vi "WPI_SPIWrite.vi"(8 "error in (no error)":errorcluster, 10 "Data To Send":u8[](array[numeric]), 11 "SPIDevRef":T1) -> (0 "error out":errorcluster, 2 "Received Data":u8[](array[numeric]), 3 "SPIDevRef":T1)   [LabVIEW 2017]
doc: "Writes data to the slave device.\n\nThis software is licensed. Open the labview\\readme\\WPI Robotics Library Open Source License.txt file for more information."
uses:
  <vilib>/Rock Robotics/WPI/SPI/WPI_SPIDevRef.ctl
  <vilib>/Rock Robotics/SystemInterfaces/spilib/spi_bus.ctl
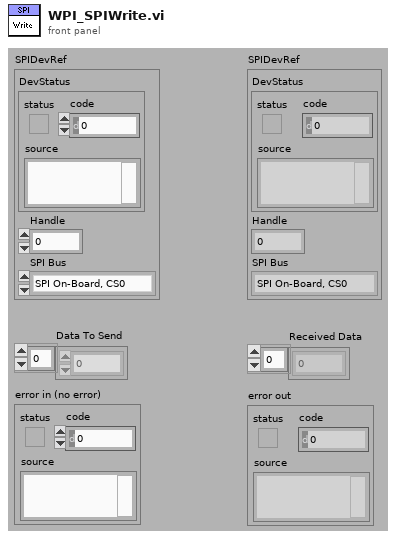
[diagram p1: front panel]
types:
  T1 = typedef "WPI_SPIDevRef.ctl" = cluster{"DevStatus":errorcluster, "Handle":i32, "SPI Bus":T2}
  T2 = typedef "spi_bus.ctl" = enum16{"SPI On-Board, CS0", "SPI On-Board, CS1", "SPI On-Board, CS2", "SPI On-Board, CS3", "SPI MXP", "Invalid"}
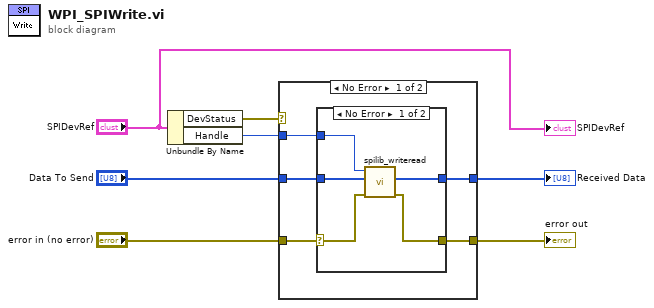
[diagram p0: block diagram]
diagram:
  n1 = Unbundle By Name("SPIDevRef") -> ("DevStatus"=w7:errorcluster, "Handle"=w3:i32)
  n2 = case shown="No Error" w7 {
    selector: w7 -> [_ w19]
    tunnel: "error in (no error)" -> [w12 _]
    tunnel: [w11 w19] -> w5
    tunnel: "Data To Send" -> [w10 _]
    tunnel: w3 -> [w9 _]
    tunnel: [w8 _] -> w2
    frame No Error {
      n3 = case shown="No Error" w12 {
        selector: w12 -> [w15 w18]
        tunnel: [w14 w18] -> w11
        tunnel: w10 -> [w16 _]
        tunnel: w9 -> [w17 _]
        tunnel: [w13 _] -> w8
        frame No Error {
          n4 = call <vilib>:"spilib_writeread.vi"("error in (no error)"=w15, "send_buf"=w16, "handle"=w17) -> ("error out"=w14:errorcluster, "recv_buf"=w13:i8[])  [unwired: 6 in, 1 out]
        }
        frame Error {
        }
      }
    }
    frame Error {
    }
  }
  "error out" <- w5
  "Received Data" <- w2
  "SPIDevRef" <- "SPIDevRef"
